vi "Experiment 25.vi"() -> ()   [LabVIEW 2026]
doc: "Experiment 25\nThis experiment (25) is like experiment 23 but uses subVIs that are distributed across two different execution systems. The subVIs in the first five loops use \"Same as caller\" (like in experiment 23), but the last 5 loops use \"Other 1\"."
uses:
  <vilib>/AdvancedString/1D String Array to Delimited String (string).vi
  <vilib>/Analysis/baseanly.llb/Mean (DBL).vi
  <vilib>/Analysis/NI_AALBase.lvlib
panel:
  out "No. Of Iterations As Block Of Text (easy to copy into Excel)":string
  out "No. Of Iterations Executed - Loop 10":i32
  out "Output - Loop 10":dbl[](array[numeric]) format="%.3f"
  out "No. Of Iterations Executed - Loop 9":i32
  out "Output - Loop 9":dbl[](array[numeric]) format="%.3f"
  out "No. Of Iterations Executed - Loop 8":i32
  out "Output - Loop 8":dbl[](array[numeric]) format="%.3f"
  out "No. Of Iterations Executed - Loop 7":i32
  out "Output - Loop 7":dbl[](array[numeric]) format="%.3f"
  out "No. Of Iterations Executed - Loop 6":i32
  out "Output - Loop 6":dbl[](array[numeric]) format="%.3f"
  out "No. Of Iterations Executed - Loop 5":i32
  out "Output - Loop 5":dbl[](array[numeric]) format="%.3f"
  out "No. Of Iterations Executed - Loop 4":i32
  out "Output - Loop 4":dbl[](array[numeric]) format="%.3f"
  out "No. Of Iterations Executed - Loop 3":i32
  out "Output - Loop 3":dbl[](array[numeric]) format="%.3f"
  out "Avg. No. Of Iterations Executed - All Loops":dbl format="%.1f"
  out "No. Of Iterations Executed - Loop 2":i32
  out "Output - Loop 2":dbl[](array[numeric]) format="%.3f"
  out "No. Of Iterations Executed - Loop 1":i32
  out "Output - Loop 1":dbl[](array[numeric]) format="%.3f"
  out "Stop VI?":bool
  # "Experiment 25"
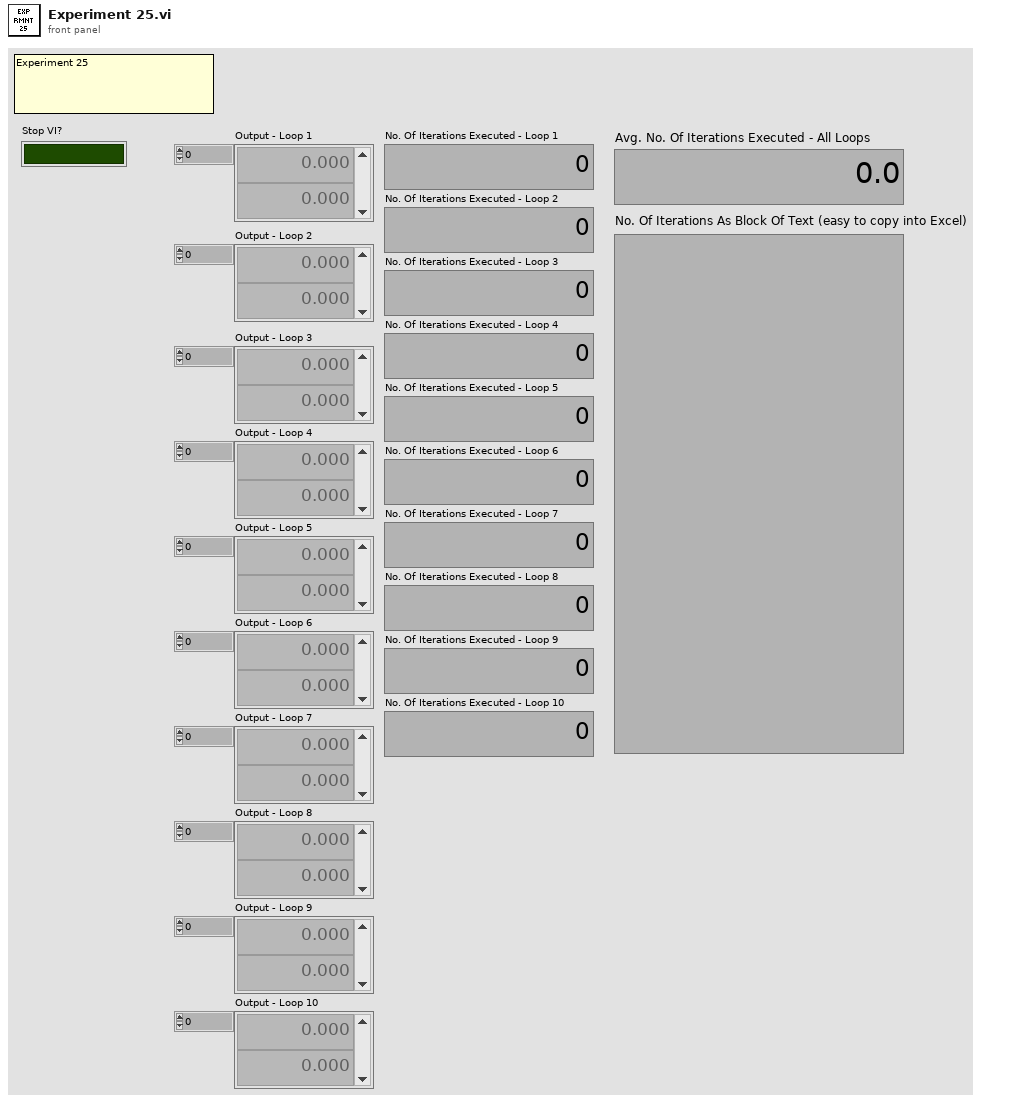
[diagram p1: front panel]
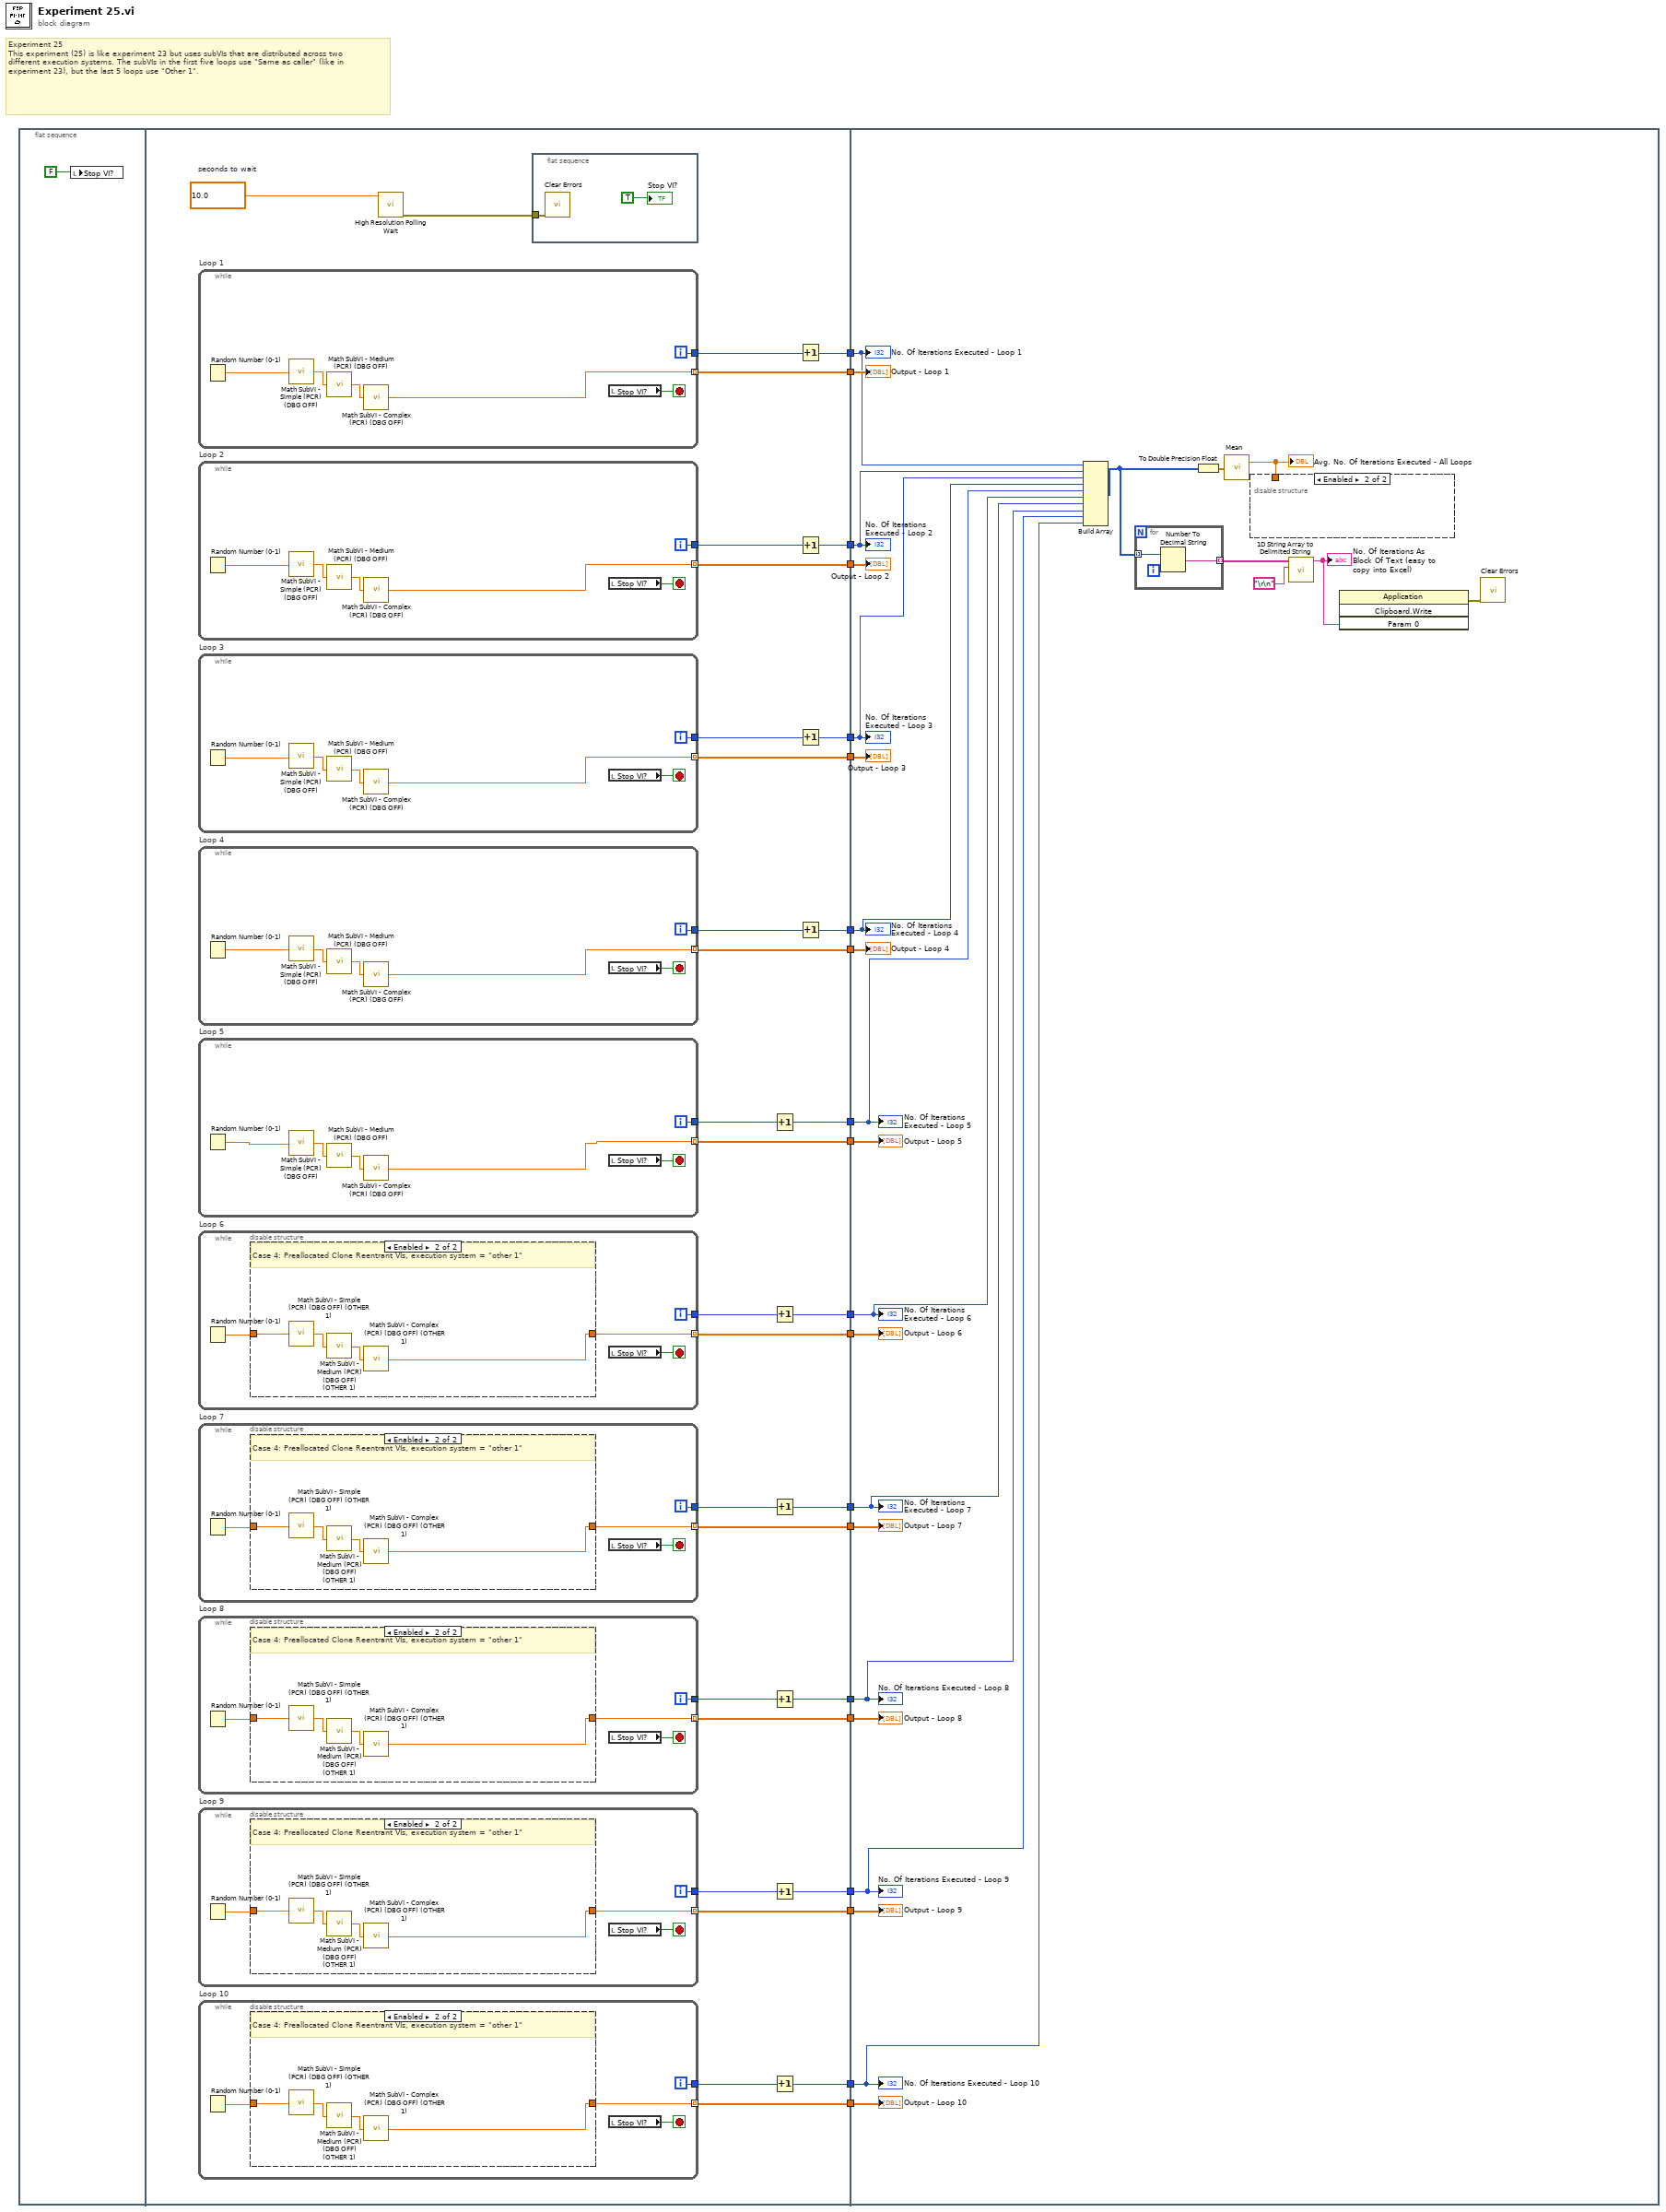
[diagram p0: block diagram]
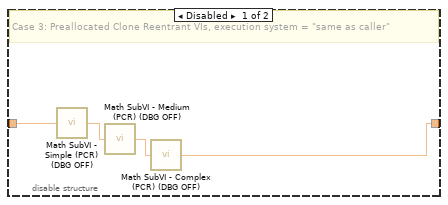
[diagram p2: hidden frame]
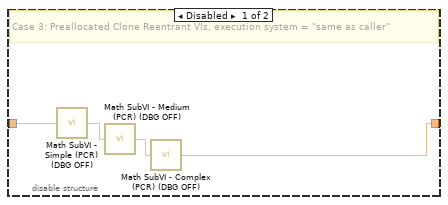
[diagram p3: hidden frame]
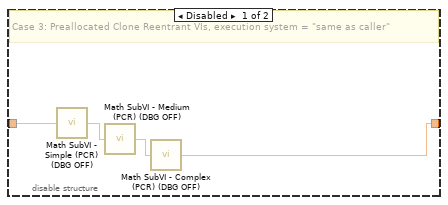
[diagram p4: hidden frame]
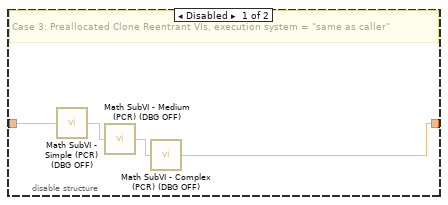
[diagram p5: hidden frame]
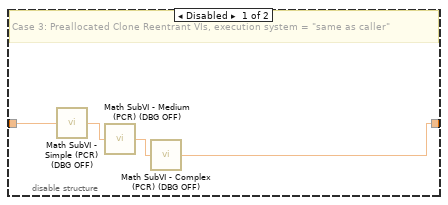
[diagram p6: hidden frame]
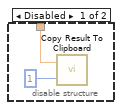
[diagram p7: hidden frame]
diagram:
  # "Experiment 25\nThis experiment (25) is like experiment 23 but uses subVIs that are distributed across two different execution systems. The subVIs in the first five loops use \"Same as caller\" (like in experiment 23), but the last 5 loops use \"Other 1\"."
  n1 = flat-sequence {
    tunnel: [w51] -> w20
    tunnel: [w49] -> w19
    tunnel: [w48] -> w18
    tunnel: [w39] -> w17
    tunnel: [w47] -> w16
    tunnel: [w37] -> w15
    tunnel: [w35] -> w14
    tunnel: [w46] -> w13
    tunnel: [w33] -> w12
    tunnel: [w45] -> w11
    tunnel: [w31] -> w10
    tunnel: [w40] -> w9
    tunnel: [w29] -> w8
    tunnel: [w41] -> w7
    tunnel: [w27] -> w6
    tunnel: [w42] -> w5
    tunnel: [w25] -> w4
    tunnel: [w43] -> w3
    tunnel: [w22] -> w2
    tunnel: [w44] -> w1
    tunnel: w20 -> [w172]
    tunnel: w19 -> [w170]
    tunnel: w18 -> [w169]
    tunnel: w17 -> [w171]
    tunnel: w16 -> [w165]
    tunnel: w15 -> [w167]
    tunnel: w14 -> [w166]
    tunnel: w13 -> [w164]
    tunnel: w12 -> [w162]
    tunnel: w11 -> [w156]
    tunnel: w10 -> [w161]
    tunnel: w9 -> [w155]
    tunnel: w8 -> [w160]
    tunnel: w7 -> [w154]
    tunnel: w6 -> [w159]
    tunnel: w5 -> [w153]
    tunnel: w4 -> [w158]
    tunnel: w3 -> [w152]
    tunnel: w2 -> [w157]
    tunnel: w1 -> [w151]
    frame #0 {
      n2 = local write "Stop VI?"(FALSE) -> ()
    }
    frame #1 {
      w53 = 10.0  # seconds to wait
      n3 = while "Loop 1" {
        tunnel: [w141] -> w51 mode=indexing
        tunnel: [w142] -> w50
        i -> [w142]
        stop <- w143 stop-if-true
        n4 = Random Number (0-1)() -> (number: 0 to 1=w140:dbl)
        n5 = call "Math SubVI - Simple (PCR) (DBG OFF).vi"("Input"=w140) -> ("Output"=w138:dbl)
        n6 = call "Math SubVI - Medium (PCR) (DBG OFF).vi"("Input"=w138) -> ("Output"=w139:dbl)
        n7 = call "Math SubVI - Complex (PCR) (DBG OFF).vi"("Input"=w139) -> ("Output"=w141:dbl)
        n8 = local read "Stop VI?"() -> (w143:bool)
      }
      n9 = while "Loop 2" {
        tunnel: [w134] -> w39 mode=indexing
        tunnel: [w136] -> w38
        i -> [w136]
        stop <- w137 stop-if-true
        n10 = Random Number (0-1)() -> (number: 0 to 1=w135:dbl)
        n11 = call "Math SubVI - Simple (PCR) (DBG OFF).vi"("Input"=w135) -> ("Output"=w132:dbl)
        n12 = call "Math SubVI - Medium (PCR) (DBG OFF).vi"("Input"=w132) -> ("Output"=w133:dbl)
        n13 = call "Math SubVI - Complex (PCR) (DBG OFF).vi"("Input"=w133) -> ("Output"=w134:dbl)
        n14 = local read "Stop VI?"() -> (w137:bool)
      }
      n15 = while "Loop 3" {
        tunnel: [w128] -> w37 mode=indexing
        tunnel: [w130] -> w36
        i -> [w130]
        stop <- w131 stop-if-true
        n16 = Random Number (0-1)() -> (number: 0 to 1=w129:dbl)
        n17 = call "Math SubVI - Simple (PCR) (DBG OFF).vi"("Input"=w129) -> ("Output"=w126:dbl)
        n18 = call "Math SubVI - Medium (PCR) (DBG OFF).vi"("Input"=w126) -> ("Output"=w127:dbl)
        n19 = call "Math SubVI - Complex (PCR) (DBG OFF).vi"("Input"=w127) -> ("Output"=w128:dbl)
        n20 = local read "Stop VI?"() -> (w131:bool)
      }
      n21 = while "Loop 4" {
        tunnel: [w122] -> w35 mode=indexing
        tunnel: [w124] -> w34
        i -> [w124]
        stop <- w125 stop-if-true
        n22 = Random Number (0-1)() -> (number: 0 to 1=w123:dbl)
        n23 = call "Math SubVI - Simple (PCR) (DBG OFF).vi"("Input"=w123) -> ("Output"=w120:dbl)
        n24 = call "Math SubVI - Medium (PCR) (DBG OFF).vi"("Input"=w120) -> ("Output"=w121:dbl)
        n25 = call "Math SubVI - Complex (PCR) (DBG OFF).vi"("Input"=w121) -> ("Output"=w122:dbl)
        n26 = local read "Stop VI?"() -> (w125:bool)
      }
      n27 = while "Loop 5" {
        tunnel: [w116] -> w33 mode=indexing
        tunnel: [w118] -> w32
        i -> [w118]
        stop <- w119 stop-if-true
        n28 = Random Number (0-1)() -> (number: 0 to 1=w117:dbl)
        n29 = call "Math SubVI - Simple (PCR) (DBG OFF).vi"("Input"=w117) -> ("Output"=w114:dbl)
        n30 = call "Math SubVI - Medium (PCR) (DBG OFF).vi"("Input"=w114) -> ("Output"=w115:dbl)
        n31 = call "Math SubVI - Complex (PCR) (DBG OFF).vi"("Input"=w115) -> ("Output"=w116:dbl)
        n32 = local read "Stop VI?"() -> (w119:bool)
      }
      n33 = while "Loop 6" {
        tunnel: [w102] -> w31 mode=indexing
        tunnel: [w104] -> w30
        i -> [w104]
        stop <- w105 stop-if-true
        n34 = Random Number (0-1)() -> (number: 0 to 1=w103:dbl)
        n35 = disable-structure shown="Enabled" {
          disable-tunnel: w103 -> [w109 w113]
          disable-tunnel: [w108 w112] -> w102
          frame Disabled {
            # "Case 3: Preallocated Clone Reentrant VIs, execution system = \"same as caller\""
            n36 = call "Math SubVI - Simple (PCR) (DBG OFF).vi"("Input"=w109) -> ("Output"=w106:dbl)
            n37 = call "Math SubVI - Medium (PCR) (DBG OFF).vi"("Input"=w106) -> ("Output"=w107:dbl)
            n38 = call "Math SubVI - Complex (PCR) (DBG OFF).vi"("Input"=w107) -> ("Output"=w108:dbl)
          }
          frame Enabled {
            # "Case 4: Preallocated Clone Reentrant VIs, execution system = \"other 1\""
            n39 = call "Math SubVI - Simple (PCR) (DBG OFF) (OTHER 1).vi"("Input"=w113) -> ("Output"=w110:dbl)
            n40 = call "Math SubVI - Medium (PCR) (DBG OFF) (OTHER 1).vi"("Input"=w110) -> ("Output"=w111:dbl)
            n41 = call "Math SubVI - Complex (PCR) (DBG OFF) (OTHER 1).vi"("Input"=w111) -> ("Output"=w112:dbl)
          }
        }
        n42 = local read "Stop VI?"() -> (w105:bool)
      }
      n43 = while "Loop 7" {
        tunnel: [w90] -> w29 mode=indexing
        tunnel: [w92] -> w28
        i -> [w92]
        stop <- w93 stop-if-true
        n44 = Random Number (0-1)() -> (number: 0 to 1=w91:dbl)
        n45 = disable-structure shown="Enabled" {
          disable-tunnel: w91 -> [w97 w101]
          disable-tunnel: [w96 w100] -> w90
          frame Disabled {
            # "Case 3: Preallocated Clone Reentrant VIs, execution system = \"same as caller\""
            n46 = call "Math SubVI - Simple (PCR) (DBG OFF).vi"("Input"=w97) -> ("Output"=w94:dbl)
            n47 = call "Math SubVI - Medium (PCR) (DBG OFF).vi"("Input"=w94) -> ("Output"=w95:dbl)
            n48 = call "Math SubVI - Complex (PCR) (DBG OFF).vi"("Input"=w95) -> ("Output"=w96:dbl)
          }
          frame Enabled {
            # "Case 4: Preallocated Clone Reentrant VIs, execution system = \"other 1\""
            n49 = call "Math SubVI - Simple (PCR) (DBG OFF) (OTHER 1).vi"("Input"=w101) -> ("Output"=w98:dbl)
            n50 = call "Math SubVI - Medium (PCR) (DBG OFF) (OTHER 1).vi"("Input"=w98) -> ("Output"=w99:dbl)
            n51 = call "Math SubVI - Complex (PCR) (DBG OFF) (OTHER 1).vi"("Input"=w99) -> ("Output"=w100:dbl)
          }
        }
        n52 = local read "Stop VI?"() -> (w93:bool)
      }
      n53 = while "Loop 8" {
        tunnel: [w78] -> w27 mode=indexing
        tunnel: [w80] -> w26
        i -> [w80]
        stop <- w81 stop-if-true
        n54 = Random Number (0-1)() -> (number: 0 to 1=w79:dbl)
        n55 = disable-structure shown="Enabled" {
          disable-tunnel: w79 -> [w85 w89]
          disable-tunnel: [w84 w88] -> w78
          frame Disabled {
            # "Case 3: Preallocated Clone Reentrant VIs, execution system = \"same as caller\""
            n56 = call "Math SubVI - Simple (PCR) (DBG OFF).vi"("Input"=w85) -> ("Output"=w82:dbl)
            n57 = call "Math SubVI - Medium (PCR) (DBG OFF).vi"("Input"=w82) -> ("Output"=w83:dbl)
            n58 = call "Math SubVI - Complex (PCR) (DBG OFF).vi"("Input"=w83) -> ("Output"=w84:dbl)
          }
          frame Enabled {
            # "Case 4: Preallocated Clone Reentrant VIs, execution system = \"other 1\""
            n59 = call "Math SubVI - Simple (PCR) (DBG OFF) (OTHER 1).vi"("Input"=w89) -> ("Output"=w86:dbl)
            n60 = call "Math SubVI - Medium (PCR) (DBG OFF) (OTHER 1).vi"("Input"=w86) -> ("Output"=w87:dbl)
            n61 = call "Math SubVI - Complex (PCR) (DBG OFF) (OTHER 1).vi"("Input"=w87) -> ("Output"=w88:dbl)
          }
        }
        n62 = local read "Stop VI?"() -> (w81:bool)
      }
      n63 = while "Loop 9" {
        tunnel: [w66] -> w25 mode=indexing
        tunnel: [w68] -> w24
        i -> [w68]
        stop <- w69 stop-if-true
        n64 = Random Number (0-1)() -> (number: 0 to 1=w67:dbl)
        n65 = disable-structure shown="Enabled" {
          disable-tunnel: w67 -> [w73 w77]
          disable-tunnel: [w72 w76] -> w66
          frame Disabled {
            # "Case 3: Preallocated Clone Reentrant VIs, execution system = \"same as caller\""
            n66 = call "Math SubVI - Simple (PCR) (DBG OFF).vi"("Input"=w73) -> ("Output"=w70:dbl)
            n67 = call "Math SubVI - Medium (PCR) (DBG OFF).vi"("Input"=w70) -> ("Output"=w71:dbl)
            n68 = call "Math SubVI - Complex (PCR) (DBG OFF).vi"("Input"=w71) -> ("Output"=w72:dbl)
          }
          frame Enabled {
            # "Case 4: Preallocated Clone Reentrant VIs, execution system = \"other 1\""
            n69 = call "Math SubVI - Simple (PCR) (DBG OFF) (OTHER 1).vi"("Input"=w77) -> ("Output"=w74:dbl)
            n70 = call "Math SubVI - Medium (PCR) (DBG OFF) (OTHER 1).vi"("Input"=w74) -> ("Output"=w75:dbl)
            n71 = call "Math SubVI - Complex (PCR) (DBG OFF) (OTHER 1).vi"("Input"=w75) -> ("Output"=w76:dbl)
          }
        }
        n72 = local read "Stop VI?"() -> (w69:bool)
      }
      n73 = while "Loop 10" {
        tunnel: [w54] -> w22 mode=indexing
        tunnel: [w56] -> w23
        i -> [w56]
        stop <- w57 stop-if-true
        n74 = Random Number (0-1)() -> (number: 0 to 1=w55:dbl)
        n75 = disable-structure shown="Enabled" {
          disable-tunnel: w55 -> [w61 w65]
          disable-tunnel: [w60 w64] -> w54
          frame Disabled {
            # "Case 3: Preallocated Clone Reentrant VIs, execution system = \"same as caller\""
            n76 = call "Math SubVI - Simple (PCR) (DBG OFF).vi"("Input"=w61) -> ("Output"=w58:dbl)
            n77 = call "Math SubVI - Medium (PCR) (DBG OFF).vi"("Input"=w58) -> ("Output"=w59:dbl)
            n78 = call "Math SubVI - Complex (PCR) (DBG OFF).vi"("Input"=w59) -> ("Output"=w60:dbl)
          }
          frame Enabled {
            # "Case 4: Preallocated Clone Reentrant VIs, execution system = \"other 1\""
            n79 = call "Math SubVI - Simple (PCR) (DBG OFF) (OTHER 1).vi"("Input"=w65) -> ("Output"=w62:dbl)
            n80 = call "Math SubVI - Medium (PCR) (DBG OFF) (OTHER 1).vi"("Input"=w62) -> ("Output"=w63:dbl)
            n81 = call "Math SubVI - Complex (PCR) (DBG OFF) (OTHER 1).vi"("Input"=w63) -> ("Output"=w64:dbl)
          }
        }
        n82 = local read "Stop VI?"() -> (w57:bool)
      }
      n83 = call <vilib>:"High Resolution Polling Wait.vi"("seconds to wait"=w53) -> ("error out"=w52:errorcluster)  [unwired: 10 in]
      n84 = flat-sequence {
        tunnel: w52 -> [w144]
        frame #0 {
          n85 = call <vilib>:"Clear Errors.vi"("error in (no error)"=w144) -> ()  [unwired: 5 in, 2 out]
          "Stop VI?" <- TRUE
        }
      }
      n86 = Increment(x=w32) -> (x+1=w45:i32)
      n87 = Increment(x=w30) -> (x+1=w40:i32)
      n88 = Increment(x=w28) -> (x+1=w41:i32)
      n89 = Increment(x=w26) -> (x+1=w42:i32)
      n90 = Increment(x=w24) -> (x+1=w43:i32)
      n91 = Increment(x=w23) -> (x+1=w44:i32)
      n92 = Increment(x=w50) -> (x+1=w49:i32)
      n93 = Increment(x=w38) -> (x+1=w48:i32)
      n94 = Increment(x=w36) -> (x+1=w47:i32)
      n95 = Increment(x=w34) -> (x+1=w46:i32)
    }
    frame #2 {
      n96 = Build Array(w170, w169, w165, w164, w156, w155, w154, w153, w152, w151) -> (w150:i32[])
      n97 = for {
        tunnel: w150 -> [w176] mode=indexing
        tunnel: [w175] -> w149 mode=indexing
        n98 = Number To Decimal String(number=w176) -> (decimal integer string=w175:string)  [unwired: 1 in]
      }
      n99 = To Double Precision Float(number=w150) -> (double precision float=w163:dbl[])
      n100 = call-poly <vilib>:"Mean.vi"("X"=w163) -> ("mean"=w168:dbl)  [unwired: 1 out]
      "Avg. No. Of Iterations Executed - All Loops" <- w168
      n101 = disable-structure shown="Enabled" {
        disable-tunnel: w168 -> [w174 _]
        frame Disabled {
          n102 = call "Copy Result To Clipboard.vi"("No. Of Decimal Places (6)"=u32 1, "Input"=w174) -> ()
        }
        frame Enabled {
        }
      }
      n103 = call-poly <vilib>:"1D String Array to Delimited String.vi"("delimiter"="\r\n", "string array"=w149) -> ("delimited string"=w146:string)  [unwired: 9 in]
      "No. Of Iterations As Block Of Text (easy to copy into Excel)" <- w146
      n104 = invoke class="Application" method="Clipboard.Write"("Param 0"=w146) -> (error out=w147:errorcluster)  [unwired: 3 in, 3 out]
      n105 = call <vilib>:"Clear Errors.vi"("error in (no error)"=w147) -> ()  [unwired: 5 in, 2 out]
      "No. Of Iterations Executed - Loop 1" <- w170
      "Output - Loop 1" <- w172
      "No. Of Iterations Executed - Loop 2" <- w169
      "Output - Loop 2" <- w171
      "No. Of Iterations Executed - Loop 3" <- w165
      "Output - Loop 3" <- w167
      "No. Of Iterations Executed - Loop 4" <- w164
      "Output - Loop 4" <- w166
      "No. Of Iterations Executed - Loop 5" <- w156
      "Output - Loop 5" <- w162
      "No. Of Iterations Executed - Loop 6" <- w155
      "Output - Loop 6" <- w161
      "No. Of Iterations Executed - Loop 7" <- w154
      "Output - Loop 7" <- w160
      "No. Of Iterations Executed - Loop 8" <- w153
      "Output - Loop 8" <- w159
      "No. Of Iterations Executed - Loop 9" <- w152
      "Output - Loop 9" <- w158
      "No. Of Iterations Executed - Loop 10" <- w151
      "Output - Loop 10" <- w157
    }
  }
